vi "Parse Event Log.vi"(6 "Log Data":string[](array[string]), 8 "error in (no error)":errorcluster, 11 "Replay in":refnum<class "Replay.lvclass">) -> (0 "error out":errorcluster, 3 "Replay out":refnum<class "Replay.lvclass">)   [LabVIEW 2016, in "CLD Exam - ATM.lvlib" / "Replay.lvclass"]
uses:
  Replay.lvclass
  Replay.lvclass/Replay.ctl
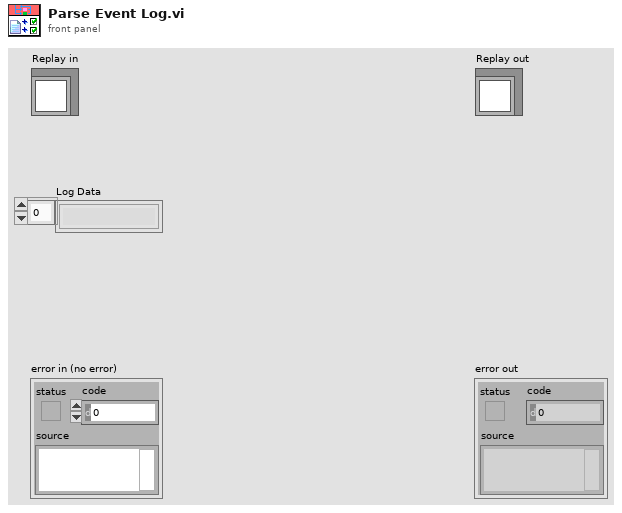
[diagram p1: front panel]
types:
  T1 = cluster{"deltaT":dbl, "Stream":string, "Name":string, "Value":string}
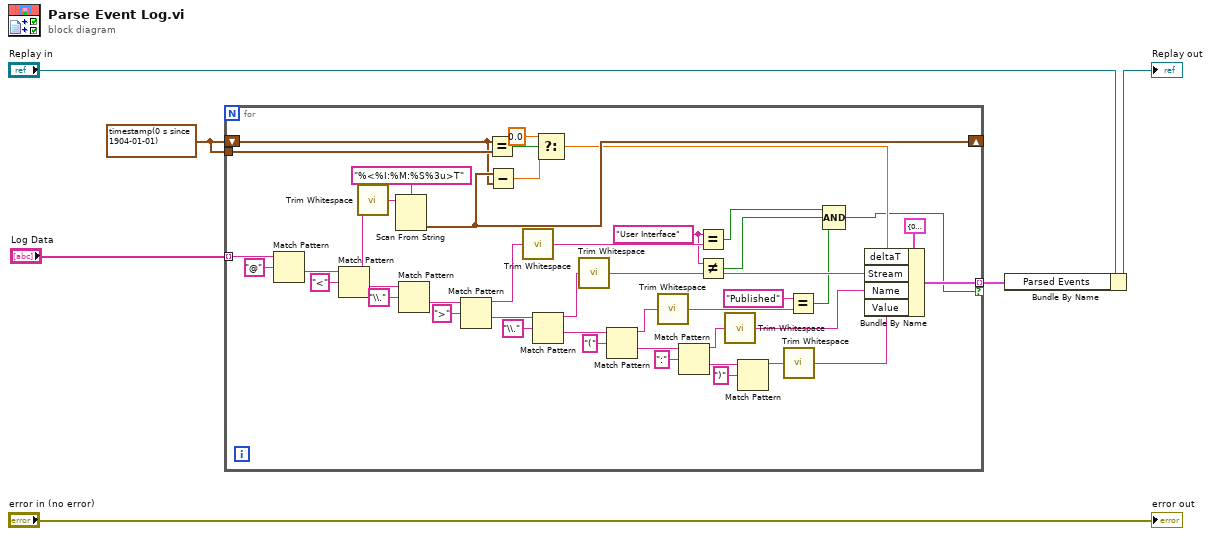
[diagram p0: block diagram]
diagram:
  w5 = timestamp(0 s since 1904-01-01) ("output 1")
  n1 = for {
    tunnel: "Log Data" -> [w50] mode=indexing
    shift-right: [w23] -> _
    shift-left: w5 -> [w22]
    tunnel: w5 -> [w26]
    tunnel: [w8] -> w1 mode=indexing if=w7
    w14 = "User Interface" ("x")
    n2 = Match Pattern(string=w50, regular expression="@") -> (after substring=w47:string)  [unwired: 1 in, 3 out]
    n3 = Match Pattern(string=w47, regular expression="<") -> (before substring=w46:string, after substring=w45:string)  [unwired: 1 in, 2 out]
    n4 = call <vilib>:"Trim Whitespace.vi"("string"=w46) -> ("trimmed string"=w28:string)  [unwired: 1 in]
    n5 = Scan From String(format string="%<%I:%M:%S%3u>T", input string=w28) -> (output 1=w23:timestamp)  [unwired: 3 in, 3 out]
    n6 = Match Pattern(string=w45, regular expression="\\.") -> (after substring=w42:string)  [unwired: 1 in, 3 out]
    n7 = Match Pattern(string=w42, regular expression=">") -> (before substring=w41:string, after substring=w39:string)  [unwired: 1 in, 2 out]
    n8 = Equal?(x=w22, y=w26) -> (x = y?=w25:bool)
    n9 = Subtract(x=w23, y=w22) -> (x-y=w21:dbl)
    n10 = call <vilib>:"Trim Whitespace.vi"("string"=w41) -> ("trimmed string"=w18:string)  [unwired: 1 in]
    n11 = Match Pattern(string=w39, regular expression="\\.") -> (before substring=w38:string, after substring=w36:string)  [unwired: 1 in, 2 out]
    n12 = Select(t=0.0, s=w25, f=w21) -> (s? t:f=w19:dbl)
    n13 = call <vilib>:"Trim Whitespace.vi"("string"=w38) -> ("trimmed string"=w15:string)  [unwired: 1 in]
    n14 = Match Pattern(string=w36, regular expression="(") -> (before substring=w35:string, after substring=w33:string)  [unwired: 1 in, 2 out]
    n15 = call <vilib>:"Trim Whitespace.vi"("string"=w35) -> ("trimmed string"=w12:string)  [unwired: 1 in]
    n16 = Match Pattern(string=w33, regular expression=":") -> (before substring=w32:string, after substring=w30:string)  [unwired: 1 in, 2 out]
    n17 = Equal?(x=w14, y=w18) -> (x = y?=w11:bool)
    n18 = Not Equal?(x=w14, y=w15) -> (x != y?=w10:bool)
    n19 = call <vilib>:"Trim Whitespace.vi"("string"=w32) -> ("trimmed string"=w17:string)  [unwired: 1 in]
    n20 = Match Pattern(string=w30, regular expression=")") -> (before substring=w29:string)  [unwired: 1 in, 3 out]
    n21 = call <vilib>:"Trim Whitespace.vi"("string"=w29) -> ("trimmed string"=w16:string)  [unwired: 1 in]
    n22 = Equal?(x="Published", y=w12) -> (x = y?=w9:bool)
    n23 = Compound Arithmetic op=AND(w11, w10, w9) -> (w7:bool)
    n24 = Bundle By Name(cluster=T1 {"deltaT"=0.0, "Stream"="", "Name"="", "Value"=""}, "deltaT"=w19, "Stream"=w15, "Name"=w17, "Value"=w16) -> (w8:T1)
  }
  n25 = Bundle By Name(cluster="Replay in", "Parsed Events"=w1) -> (→"Replay out":refnum<class "Replay.lvclass">)
  "error out" <- "error in (no error)"
